vi "Oven_LOG_test.vi"() -> ()   [LabVIEW 2017]
uses:
  <vilib>/addons/database/Connection.llb/DB Tools Open Connec (Path).vi
  <vilib>/addons/database/NI_Database_API.lvlib
panel:
  in  "DATE":string
  out "data":variant
  out "error out":errorcluster
  in  "PRESSURE_2nd":string
  in  "PRESSURE_1st":string
  in  "HOLDING_TIME":string
  in  "MR_RETURN_TIME":string
  in  "Heating_time":string
  in  "Bottom_zone_8":string
  in  "Bottom_zone_7":string
  in  "Bottom_zone_6":string
  in  "Bottom_zone_5":string
  in  "Bottom_zone_4":string
  in  "Bottom_zone_3":string
  in  "Bottom_zone_2":string
  in  "Bottom_zone_1":string
  in  "Top_zone_8":string
  in  "Top_zone_7":string
  in  "Top_zone_6":string
  in  "Top_zone_5":string
  in  "Top_zone_4":string
  in  "Top_zone_3":string
  in  "Top_zone_2":string
  in  "Top_zone_1":string
  in  "PRODUCT_CODE":string
  in  "PLAN_DATE":string
  in  "SHIFT":i32
  in  "STATION_ID":string
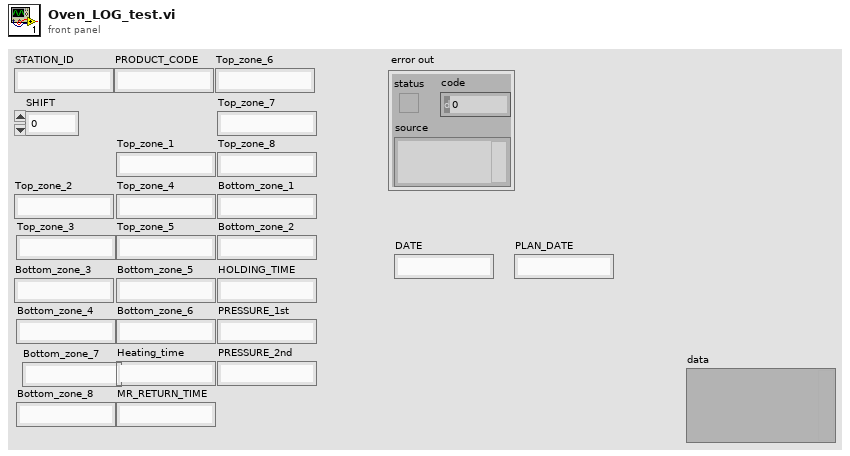
[diagram p1: front panel]
types:
  T1 = cluster{"STATION_ID":string, "DATE":string, "SHIFT":string, "PLAN_DATE":string, "PRODUCT_CODE":string, "Top_zone_1":string, "Top_zone_2":string, "Top_zone_3":string, "Top_zone_4":string, "Top_zone_5":string, "Top_zone_6":string, "Top_zone_7":string, "Top_zone_8":string, "Bottom_zone_1":string, "Bottom_zone_2":string, "Bottom_zone_3":string, "Bottom_zone_4":string, "Bottom_zone_5":string, "Bottom_zone_6":string, "Bottom_zone_7":string, "Bottom_zone_8":string, "Heating_time":string, "MR_RETURN_TIME":string, "HOLDING_TIME":string, "PRESSURE_1st":string, "PRESSURE_2nd":string}
  T2 = typedef "NI_Database_API.lvlib/Conn ObjectReference.ctl" = refnum<k1>
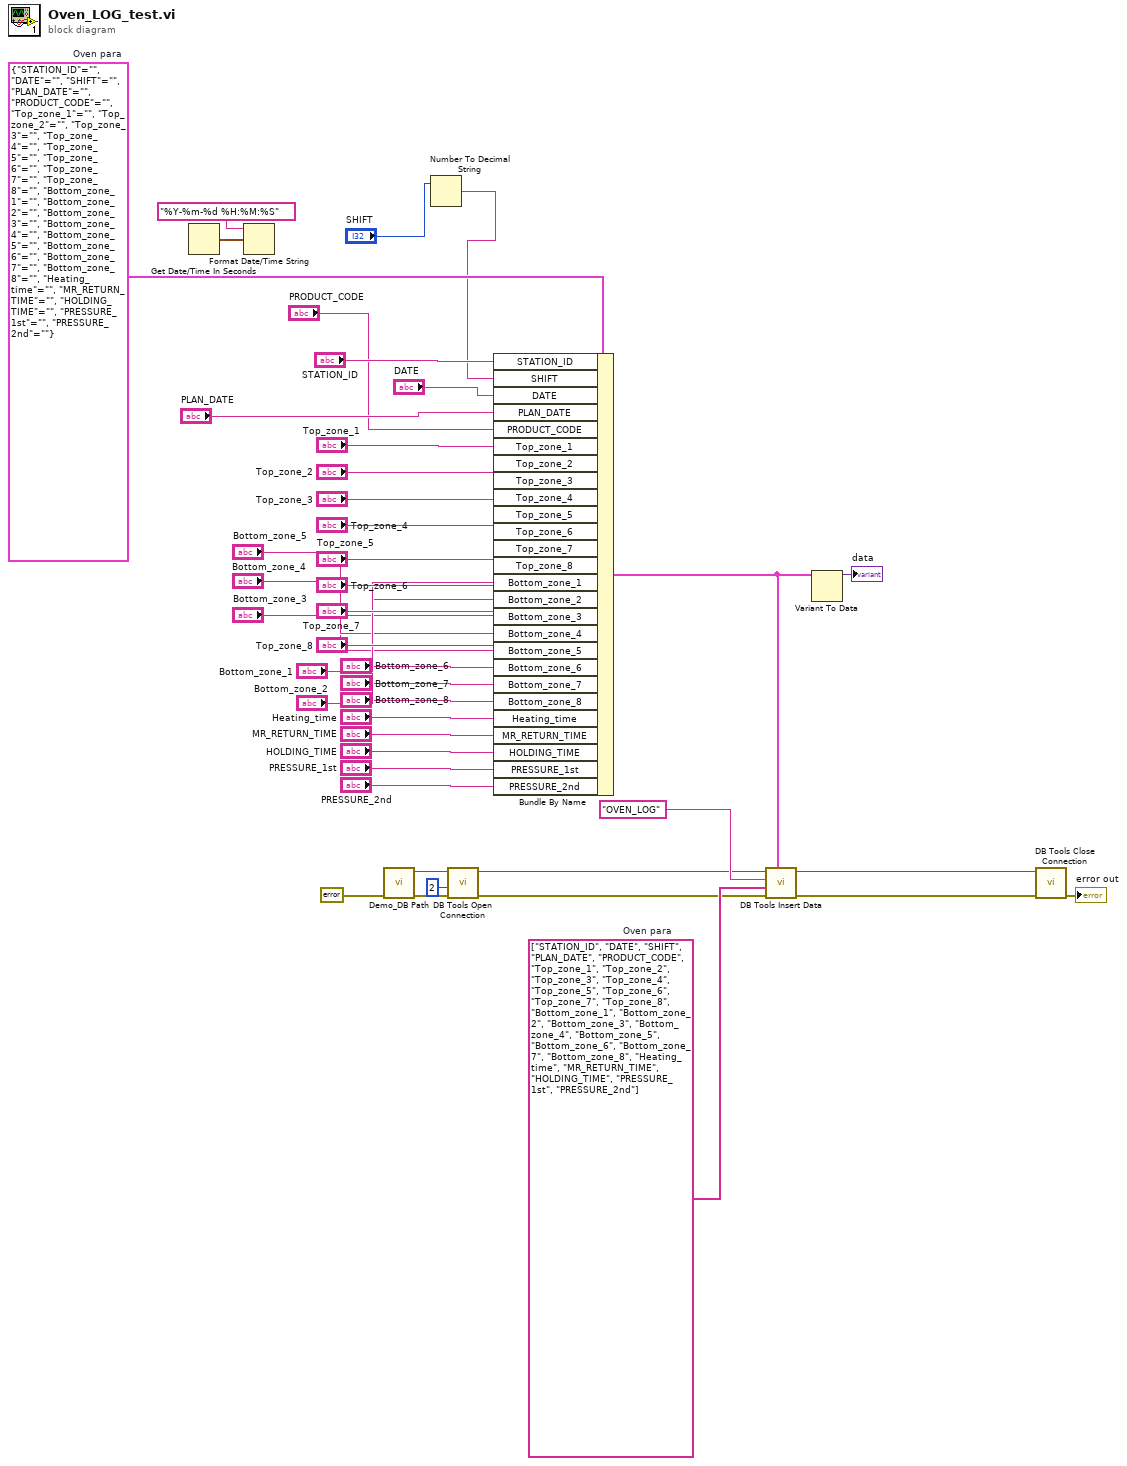
[diagram p0: block diagram]
diagram:
  w33 = T1 {"STATION_ID"="", "DATE"="", "SHIFT"="", "PLAN_DATE"="", "PRODUCT_CODE"="", "Top_zone_1"="", "Top_zone_2"="", "Top_zone_3"="", "Top_zone_4"="", "Top_zone_5"="", "Top_zone_6"="", "Top_zone_7"="", "Top_zone_8"="", "Bottom_zone_1"="", "Bottom_zone_2"="", "Bottom_zone_3"="", "Bottom_zone_4"="", "Bottom_zone_5"="", "Bottom_zone_6"="", "Bottom_zone_7"="", "Bottom_zone_8"="", "Heating_time"="", "MR_RETURN_TIME"="", "HOLDING_TIME"="", "PRESSURE_1st"="", "PRESSURE_2nd"=""}  # Oven para
  w42 = string[] ["STATION_ID", "DATE", "SHIFT", "PLAN_DATE", "PRODUCT_CODE", "Top_zone_1", "Top_zone_2", "Top_zone_3", "Top_zone_4", "Top_zone_5", "Top_zone_6", "Top_zone_7", "Top_zone_8", "Bottom_zone_1", "Bottom_zone_2", "Bottom_zone_3", "Bottom_zone_4", "Bottom_zone_5", "Bottom_zone_6", "Bottom_zone_7", "Bottom_zone_8", "Heating_time", "MR_RETURN_TIME", "HOLDING_TIME", "PRESSURE_1st", "PRESSURE_2nd"]  # Oven para
  n1 = Get Date/Time In Seconds() -> (seconds since 1Jan1904=w6:timestamp)
  n2 = Format Date/Time String(time format string (%c)="%Y-%m-%d %H:%M:%S", seconds (now)=w6) -> ()  [unwired: 1 in, 1 out]
  n3 = call "Demo_DB Path.vi"("error in"=errorcluster {"status"=FALSE, "code"=0, "source"=""} ("error constant")) -> ("error out"=w41:errorcluster, "DB Path"=w40:path)  [unwired: 9 in]
  n4 = Number To Decimal String(number="SHIFT") -> (decimal integer string=w2:string)  [unwired: 1 in]
  n5 = call-poly <vilib>:"DB Tools Open Connection.vi"("error in (no error)"=w41, "connection timeout (15)"=2, "connection information"=w40) -> ("error out"=w36:errorcluster, "connection reference"=w37:T2)  [unwired: 5 in]
  n6 = Bundle By Name(cluster=w33, "STATION_ID"="STATION_ID", "SHIFT"=w2, "DATE"="DATE", "PLAN_DATE"="PLAN_DATE", "PRODUCT_CODE"="PRODUCT_CODE", "Top_zone_1"="Top_zone_1", "Top_zone_2"="Top_zone_2", "Top_zone_3"="Top_zone_3", "Top_zone_4"="Top_zone_4", "Top_zone_5"="Top_zone_5", "Top_zone_6"="Top_zone_6", "Top_zone_7"="Top_zone_7", "Top_zone_8"="Top_zone_8", "Bottom_zone_1"="Bottom_zone_1", "Bottom_zone_2"="Bottom_zone_2", "Bottom_zone_3"="Bottom_zone_3", "Bottom_zone_4"="Bottom_zone_4", "Bottom_zone_5"="Bottom_zone_5", "Bottom_zone_6"="Bottom_zone_6", "Bottom_zone_7"="Bottom_zone_7", "Bottom_zone_8"="Bottom_zone_8", "Heating_time"="Heating_time", "MR_RETURN_TIME"="MR_RETURN_TIME", "HOLDING_TIME"="HOLDING_TIME", "PRESSURE_1st"="PRESSURE_1st", "PRESSURE_2nd"="PRESSURE_2nd") -> (w5:T1)
  n7 = call <vilib>:"DB Tools Insert Data.vi"("data"=w5, "error in (no error)"=w36, "columns"=w42, "table"="OVEN_LOG", "connection reference"=w37) -> ("error out"=w34:errorcluster, "connection reference out"=w35:T2)  [unwired: 5 in]
  n8 = Variant To Data(Variant=w5) -> (data=→"data":variant)  [unwired: 2 in, 1 out]
  n9 = call <vilib>:"DB Tools Close Connection.vi"("error in (no error)"=w34, "connection reference"=w35) -> ("error out"=→"error out":errorcluster)  [unwired: 5 in]
